vi "CohortWFM.vi"(8 "error in (no error)":errorcluster, 10 "Sampling Frequency [Hz]":u32 format="%.2p", 11 "Cohort in":refnum<class "Cohort.lvclass">) -> (0 "error out":errorcluster, 1 "Cohort Signal":dbl[](array[numeric]), 2 "dt":sgl, 3 "Cohort out":refnum<class "Cohort.lvclass">)   [LabVIEW 2012, in "Cohort.lvclass"]
uses:
  Cohort.lvclass
  Electrode.lvclass
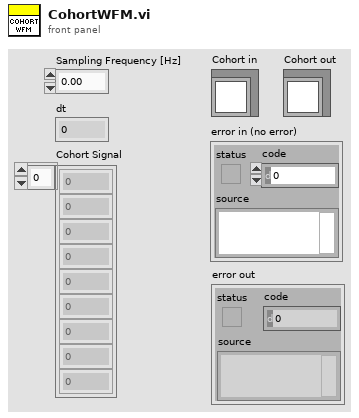
[diagram p1: front panel]
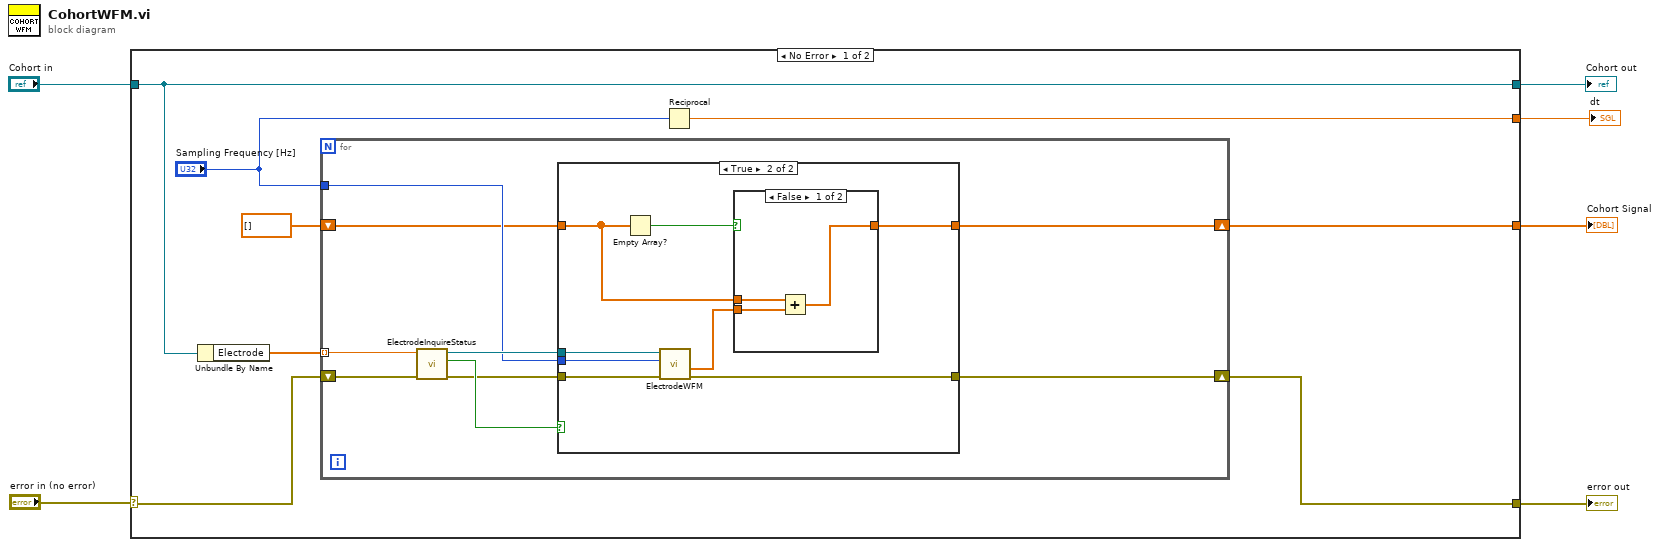
[diagram p0: block diagram]
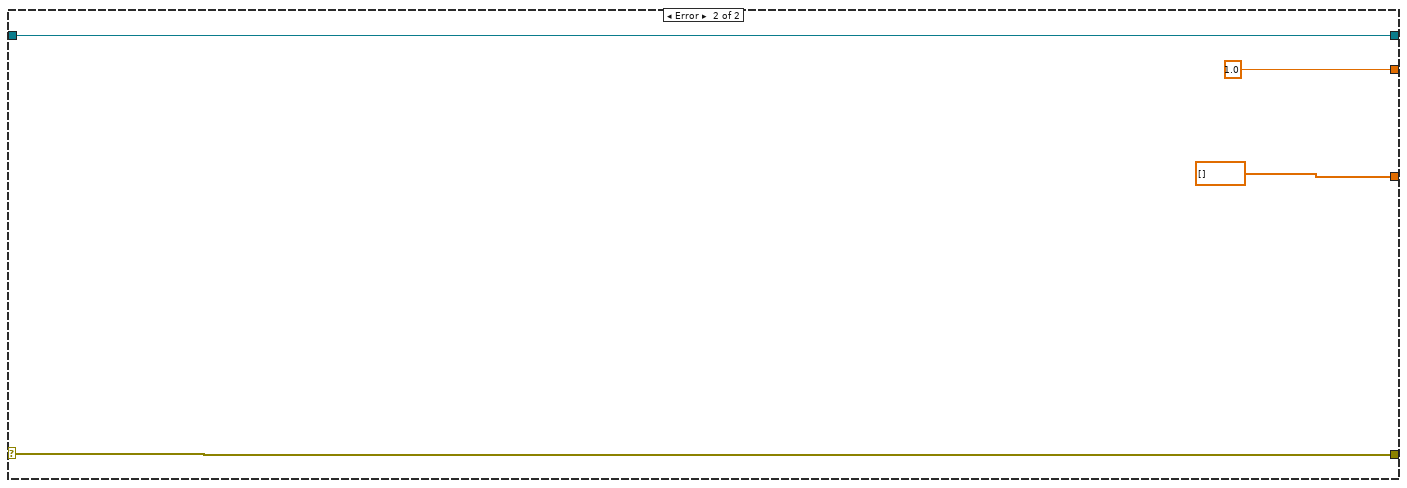
[diagram p4: hidden frame]
diagram:
  n1 = case shown="No Error" "error in (no error)" {
    selector: "error in (no error)" -> [w9 w40]
    tunnel: [w8 w40] -> w5
    tunnel: [w14 w41] -> w3
    tunnel: "Cohort in" -> [w14 w41]
    tunnel: [w12 dbl[] [] ("Signal Array")] -> w2
    tunnel: [w11 1.0] -> w1
    frame No Error {
      n2 = Unbundle By Name(w14) -> ("Electrode"=w13:sgl[])
      n3 = for {
        tunnel: w13 -> [w23] mode=indexing
        shift-right: [w17] -> w12
        shift-left: dbl[] [] ("Signal Array") -> [w18]
        tunnel: "Sampling Frequency [Hz]" -> [w19]
        shift-right: [w16] -> w8
        shift-left: w9 -> [w15]
        n4 = call-dynamic "ElectrodeInquireStatus.vi"("error in (no error)"=w15, "Electrode in"=w23) -> ("error out"=w21:errorcluster, "Electrode Activated?"=w22:bool, "Electrode out"=w20:refnum<class "Electrode.lvclass">)  [unwired: 7 in]
        n5 = case shown="True" w22 {
          tunnel: w21 -> [w25 w32]
          tunnel: w20 -> [_ w33]
          tunnel: [w25 w31] -> w16
          tunnel: w19 -> [_ w30]
          tunnel: w18 -> [w24 w26]
          tunnel: [w24 w27] -> w17
          frame False {
          }
          frame True {
            n6 = Empty Array?(array=w26) -> (empty?=w29:bool)
            n7 = call "ElectrodeWFM.vi"("Electrode in"=w33, "Sampling Rate [Hz]"=w30, "error in (no error)"=w32) -> ("Signal Array"=w28:dbl[], "error out"=w31:errorcluster)  [unwired: 3 in, 3 out]
            n8 = case shown="False" w29 {
              tunnel: w28 -> [w36 w37]
              tunnel: [w34 w37] -> w27
              tunnel: w26 -> [w35 _]
              frame False {
                n9 = Add(x=w35, y=w36) -> (x+y=w34:dbl[])
              }
              frame True {
              }
            }
          }
        }
      }
      n10 = Reciprocal(x="Sampling Frequency [Hz]") -> (1/x=w11:dbl)
    }
    frame Error {
    }
  }
  "error out" <- w5
  "Cohort out" <- w3
  "Cohort Signal" <- w2
  "dt" <- w1
